vi "HEWH MW100 DAQ Data Notifier.vi"(7 "Status":T2, 8 "error in (no error)":errorcluster, 10 "Set Status":T1={"Voltage (Volts)"=236.2, "Current (Amps)"=17.749, "Power (Watts)"=4192.0, "WattHours (Wh)"=0.0, "TC Tree (AVG)"=0.0, "Flow Rate (GPM)"=0.0, "Gallons (Gal)"=0.0, "RTD Out (Deg F)"=0.0, "TC Down"=0.0, "TC Tree Array"=[], "UE Event Lead"=0, "LE Event Lead"=0}, 11 "name (unnamed)":string) -> (0 "error out":errorcluster, 3 "latest notification":T1={"Voltage (Volts)"=236.2, "Current (Amps)"=17.749, "Power (Watts)"=4192.0, "WattHours (Wh)"=0.0, "TC Tree (AVG)"=0.0, "Flow Rate (GPM)"=0.0, "Gallons (Gal)"=0.0, "RTD Out (Deg F)"=0.0, "TC Down"=0.0, "TC Tree Array"=[], "UE Event Lead"=0, "LE Event Lead"=0})   [LabVIEW 2014]
uses:
  Utility/Type Definitions/UTILITY Notifier.ctl
  Type Definitions/HEWH Power Data.ctl
panel:
  in  "DAQ (Data Type)":T1={"Voltage (Volts)"=236.2, "Current (Amps)"=17.749, "Power (Watts)"=4192.0, "WattHours (Wh)"=0.0, "TC Tree (AVG)"=0.0, "Flow Rate (GPM)"=0.0, "Gallons (Gal)"=0.0, "RTD Out (Deg F)"=0.0, "TC Down"=0.0, "TC Tree Array"=[], "UE Event Lead"=0, "LE Event Lead"=0}
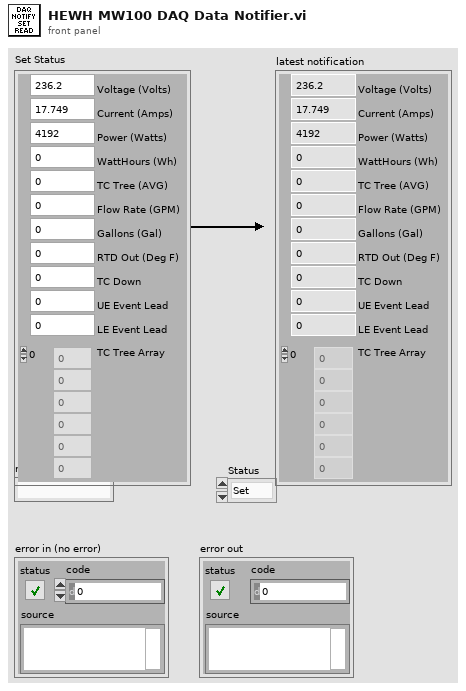
[diagram p1: front panel]
types:
  T1 = typedef "HEWH Power Data.ctl" = cluster{"Voltage (Volts)":dbl, "Current (Amps)":dbl, "Power (Watts)":dbl, "WattHours (Wh)":dbl, "TC Tree (AVG)":dbl, "Flow Rate (GPM)":dbl, "Gallons (Gal)":dbl, "RTD Out (Deg F)":dbl, "TC Down":dbl, "TC Tree Array":dbl[], "UE Event Lead":i32, "LE Event Lead":i32}
  T2 = typedef "UTILITY Notifier.ctl" = enum16{"Set", "Read", "Release Ref"}
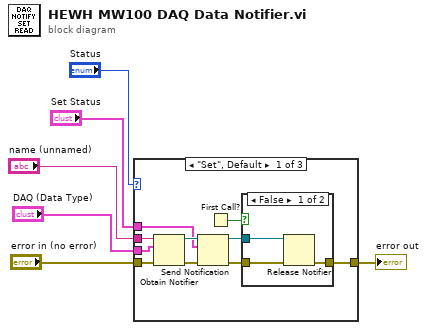
[diagram p0: block diagram]
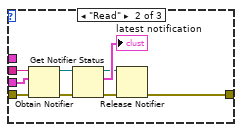
[diagram p3: hidden frame]
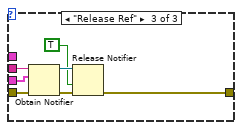
[diagram p4: hidden frame]
diagram:
  n1 = case shown="\"Set\", Default" "Status" {
    tunnel: [w7 w21 w30] -> w6
    tunnel: "error in (no error)" -> [w14 w27 w36]
    tunnel: "name (unnamed)" -> [w13 w26 w33]
    tunnel: "DAQ (Data Type)" -> [w11 w25 w32]
    tunnel: "Set Status" -> [w12 _ _]
    frame "Set", Default {
      n2 = Obtain Notifier(name (unnamed)=w13, notification data type=w11, error in (no error)=w14) -> (notifier out=w15:refnum<notifier>, error out=w16:errorcluster)  [unwired: 1 in, 1 out]
      n3 = Send Notification(notification=w12, notifier=w15, error in (no error)=w16) -> (notifier out=w8:refnum<notifier>, error out=w9:errorcluster)
      n4 = First Call?() -> (First Call?: T/F=w10:bool)
      n5 = case shown="False" w10 {
        tunnel: w9 -> [w18 w20]
        tunnel: w8 -> [w19 _]
        tunnel: [w17 w20] -> w7
        frame False {
          n6 = Release Notifier(notifier=w19, error in (no error)=w18) -> (error out=w17:errorcluster)  [unwired: 1 in, 2 out]
        }
        frame True {
        }
      }
    }
    frame "Read" {
      n7 = Obtain Notifier(name (unnamed)=w26, notification data type=w25, error in (no error)=w27) -> (notifier out=w28:refnum<notifier>, error out=w29:errorcluster)  [unwired: 1 in, 1 out]
      n8 = Get Notifier Status(notifier=w28, error in (no error)=w29) -> (notifier out=w23:refnum<notifier>, current notification=→"latest notification":T1, error out=w22:errorcluster)  [unwired: 2 out]
      n9 = Release Notifier(notifier=w23, error in (no error)=w22) -> (error out=w21:errorcluster)  [unwired: 1 in, 2 out]
    }
    frame "Release Ref" {
      n10 = Obtain Notifier(name (unnamed)=w33, notification data type=w32, error in (no error)=w36) -> (notifier out=w34:refnum<notifier>, error out=w35:errorcluster)  [unwired: 1 in, 1 out]
      n11 = Release Notifier(notifier=w34, force destroy? (F)=TRUE, error in (no error)=w35) -> (error out=w30:errorcluster)  [unwired: 2 out]
    }
  }
  "error out" <- w6
